vi "convert cell pair to dbl.vi"(8 "error in":errorcluster, 10 "start index":i32=6, 11 "Array":string[](array[string])) -> (0 "error out":errorcluster, 2 "Numeric of start index +1":dbl, 3 "Numeric of start index":dbl)   [LabVIEW 2016]
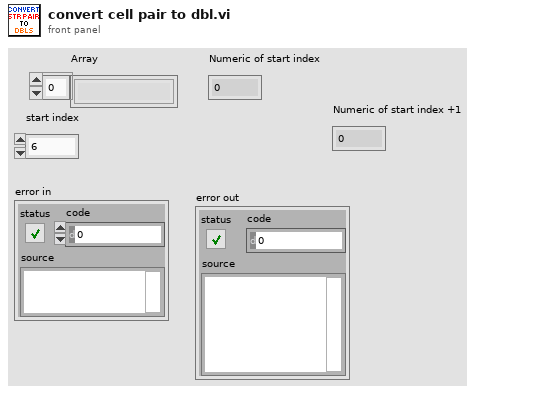
[diagram p1: front panel]
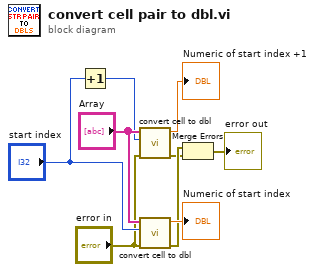
[diagram p0: block diagram]
diagram:
  n1 = Increment(x="start index") -> (x+1=w5:i32)
  n2 = call "convert cell to dbl.vi"("error in"="error in", "start index"=w5, "Array"="Array") -> ("error out"=w2:errorcluster, "Numeric of start index"=→"Numeric of start index +1":dbl)  [unwired: 7 in]
  n3 = call "convert cell to dbl.vi"("error in"="error in", "start index"="start index", "Array"="Array") -> ("error out"=w8:errorcluster, "Numeric of start index"=→"Numeric of start index":dbl)  [unwired: 7 in]
  n4 = Merge Errors(w8, w2) -> (→"error out":errorcluster)
